vi "Radians to Degrees (Scalar DBL).vi"(3 "angle (rad)":dbl) -> (1 "angle (deg)":dbl)   [LabVIEW 2020, in "NI_AngleManipulation.lvlib"]
doc: "Converts an angle from radians to degrees."
uses:
  <vilib>/Utility/AngleManip/NI_AngleManipulation.lvlib
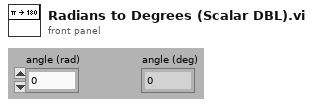
[diagram p1: front panel]
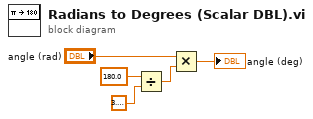
[diagram p0: block diagram]
diagram:
  n1 = Divide(x=180.0 ("y"), y=3.141592653589793) -> (x/y=w2:dbl)
  n2 = Multiply(x="angle (rad)", y=w2) -> (x*y=→"angle (deg)":dbl)
